vi "Pos ctrl window-Queue interface.vi"(10 "Function":enum16{"None", "Release queue", "Obtain queue"}(ring)) -> (0 "error out":errorcluster, 3 "Pos ctrl window queue":refnum<queue>)   [LabVIEW 2020]
uses:
  Typedefs/Pos Ctrl queue data cluster.ctl
  Typedefs/Pos Ctrl States.ctl
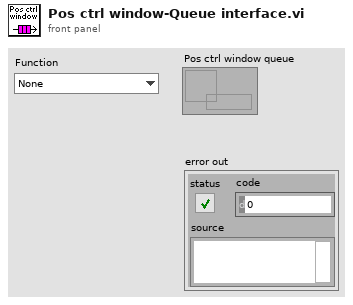
[diagram p1: front panel]
types:
  T1 = typedef "Pos Ctrl queue data cluster.ctl" = cluster{"State":T2, "variant":variant}
  T2 = typedef "Pos Ctrl States.ctl" = enum16{"Idle", "Count-down", "Request single step (ack.)", "Request single step (no ack.)", "Request continuous movement", "Request movement stop"}
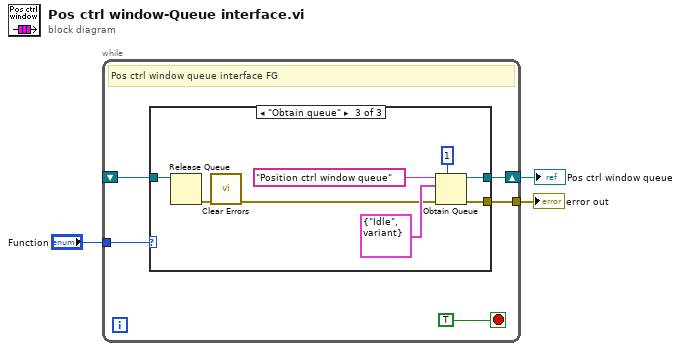
[diagram p0: block diagram]
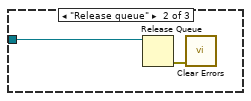
[diagram p3: hidden frame]
diagram:
  n1 = while {
    shift-right: [w7] -> w3
    shift-left: _ -> [w5]
    tunnel: "Function" -> [w6]
    tunnel: [w4] -> w1
    stop <- TRUE stop-if-true
    # "Pos ctrl window queue interface FG"
    n2 = case shown="\"Obtain queue\"" w6 {
      tunnel: w5 -> [w9 w11 w19]
      tunnel: [w9 _ w14] -> w7
      tunnel: [_ _ w12] -> w4
      frame "None", Default {
      }
      frame "Release queue" {
        n3 = Release Queue(queue=w11) -> (error out=w10:errorcluster)  [unwired: 2 in, 2 out]
        n4 = call <vilib>:"Clear Errors.vi"("error in (no error)"=w10) -> ()  [unwired: 5 in, 2 out]
      }
      frame "Obtain queue" {
        n5 = Release Queue(queue=w19) -> (error out=w18:errorcluster)  [unwired: 2 in, 2 out]
        n6 = call <vilib>:"Clear Errors.vi"("error in (no error)"=w18) -> ("error out"=w13:errorcluster)  [unwired: 5 in, 1 out]
        n7 = Obtain Queue(max queue size (-1, unlimited)=1, name (unnamed)="Position ctrl window queue", element data type=T1 {"State"=enum."Idle", "variant"=variant} ("Pos Ctrl queue data cluster"), error in (no error)=w13) -> (queue out=w14:refnum<queue>, error out=w12:errorcluster)  [unwired: 1 in, 1 out]
      }
    }
  }
  "Pos ctrl window queue" <- w3
  "error out" <- w1
